vi "Search for Channel Data Reference.vi"(8 "error in (no error)":errorcluster, 9 "Access":T2, 10 "Item Ref":T1 format="%.0x", 11 "Device Ref in":T1=18446744073709551615 format="%.0x") -> (0 "error out":errorcluster, 3 "Channel Data Reference":T3 format="%.0x")   [LabVIEW 2017, in "Ballard MIL-1553 Engine.lvlib"]
uses:
  <vilib>/NI Veristand/Custom Device API/Data Reference.ctl
  <vilib>/NI Veristand/Custom Device API/Custom Device Item Ref.ctl
  <vilib>/NI Veristand/Custom Device API/Data Access Type.ctl
  Ballard MIL-1553 Engine.lvlib
  <vilib>/NI VeriStand/Custom Device API/Custom Device API.lvlib
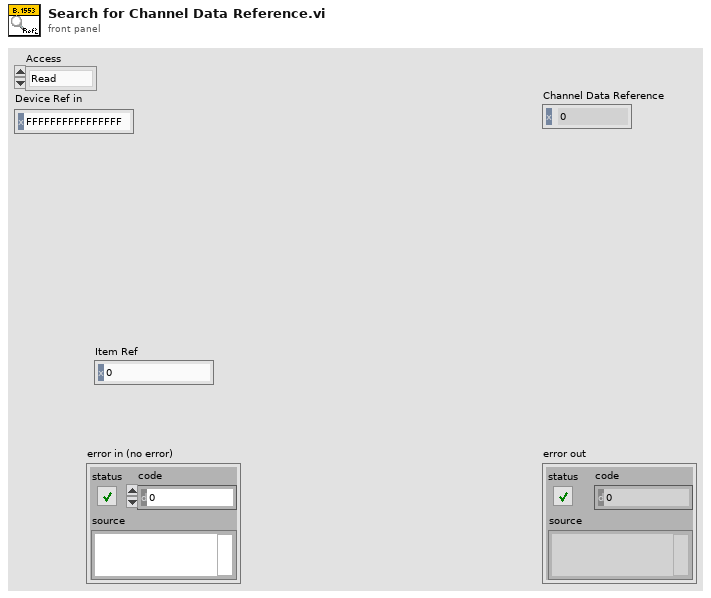
[diagram p1: front panel]
types:
  T1 = typedef "Custom Device API.lvlib/Custom Device Item Ref.ctl" = u64
  T2 = typedef "Custom Device API.lvlib/Data Access Type.ctl" = enum16{"Read", "Write"}
  T3 = typedef "Custom Device API.lvlib/Data Reference.ctl" = i32
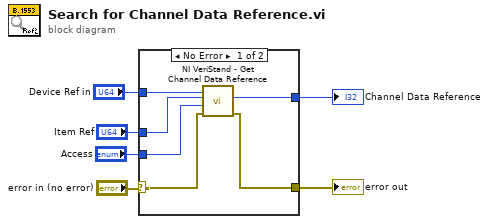
[diagram p0: block diagram]
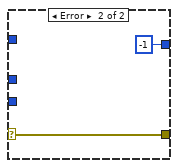
[diagram p2: hidden frame]
diagram:
  n1 = case shown="No Error" "error in (no error)" {
    selector: "error in (no error)" -> [w11 w14]
    tunnel: [w10 w14] -> w5
    tunnel: [w12 -1 ("index of element")] -> w4
    tunnel: "Item Ref" -> [w9 _]
    tunnel: "Access" -> [w8 _]
    tunnel: "Device Ref in" -> [w7 _]
    frame No Error {
      n2 = call <vilib>:"NI VeriStand - Get Channel Data Reference.vi"("error in (no error)"=w11, "Access"=w8, "Channel Ref in"=w9, "Device Ref in"=w7) -> ("error out"=w10:errorcluster, "Channel Data Reference"=w12:T3)  [unwired: 5 in, 1 out]
    }
    frame Error {
    }
  }
  "error out" <- w5
  "Channel Data Reference" <- w4
